vi "Response hndler.vi"(10 "Recived MSG":string, 11 "Domino LM.lvlib:Domino Laser module Class.lvclass":refnum<class "Domino Laser module Class.lvclass">) -> (1 "Command Excuted successfully?":bool, 2 "printer response":string, 3 "Domino LM.lvlib:Domino Laser module Class.lvclass 2":refnum<class "Domino Laser module Class.lvclass">)   [LabVIEW 2024, in "Domino LM.lvlib" / "Domino Laser module Class.lvclass"]
uses:
  CTRLS/Domino Laser module Class.lvclass
  <vilib>/Utility/error.llb/Trim Whitespace One-Sided.vi
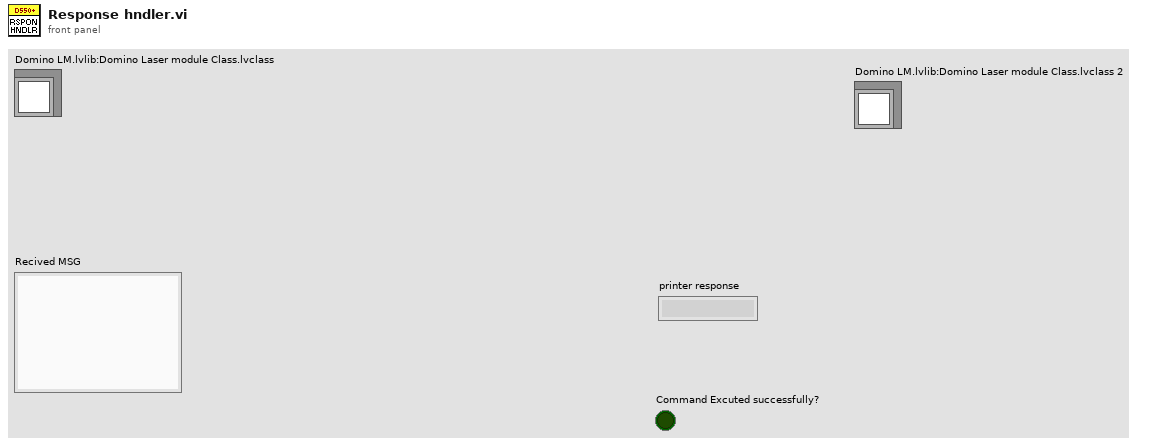
[diagram p1: front panel]
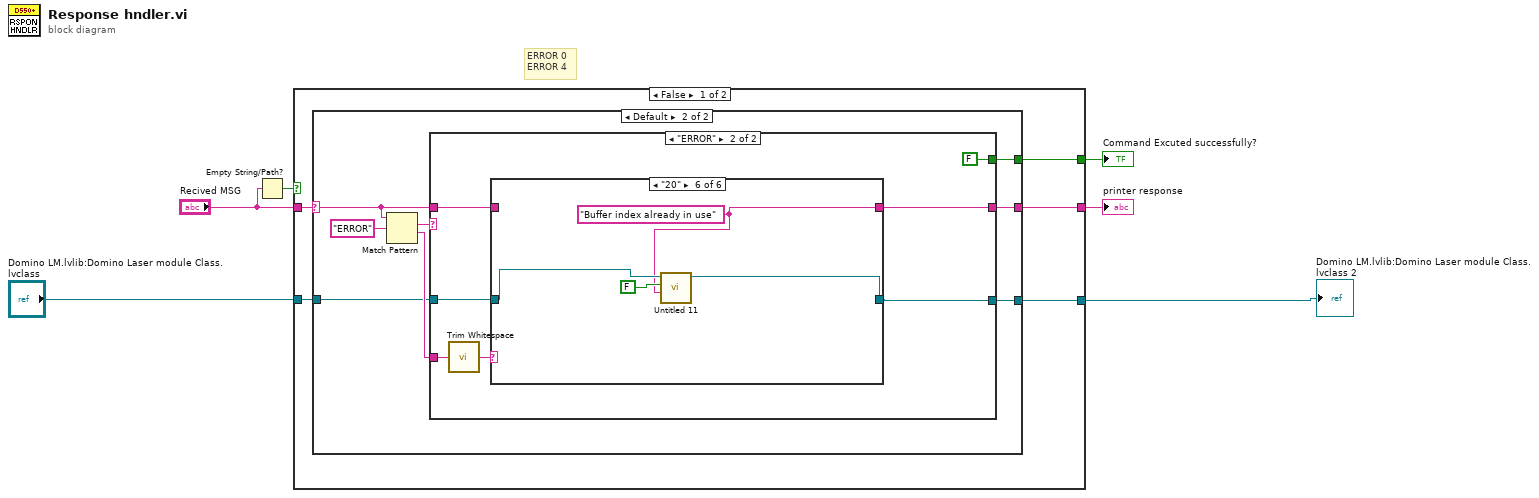
[diagram p0: block diagram]
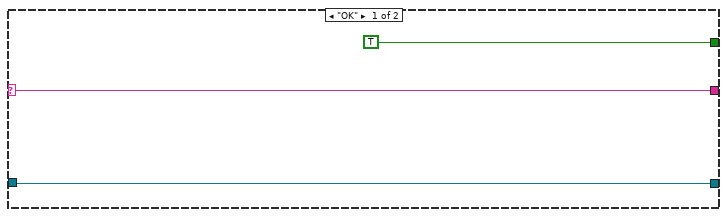
[diagram p2: hidden frame]
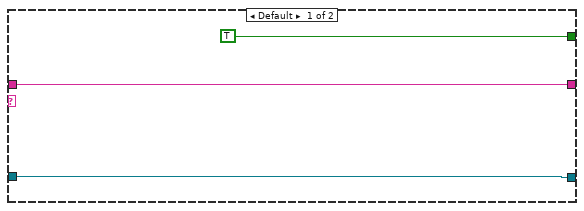
[diagram p3: hidden frame]
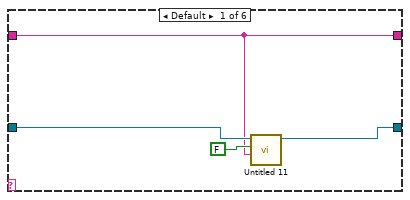
[diagram p4: hidden frame]
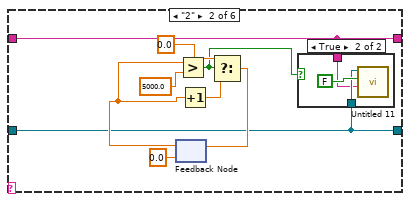
[diagram p5: hidden frame]
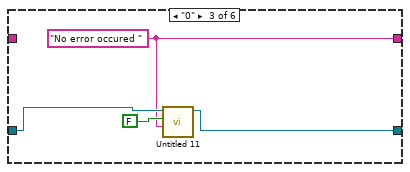
[diagram p7: hidden frame]
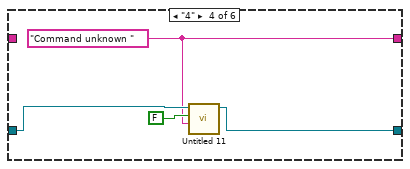
[diagram p8: hidden frame]
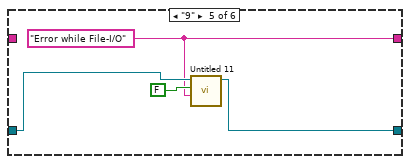
[diagram p9: hidden frame]
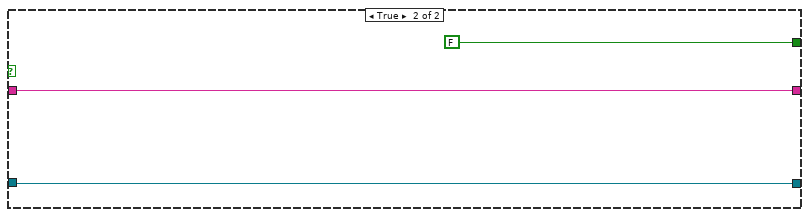
[diagram p10: hidden frame]
diagram:
  # "ERROR 0\nERROR 4"
  n1 = Empty String/Path?(string/path="Recived MSG") -> (empty?=w3:bool)
  n2 = case shown="False" w3 {
    tunnel: "Recived MSG" -> [w11 w66]
    tunnel: [w10 FALSE] -> w6
    tunnel: [w9 w66] -> w5
    tunnel: "Domino LM.lvlib:Domino Laser module Class.lvclass" -> [w8 w65]
    tunnel: [w7 w65] -> w1
    frame False {
      n3 = case shown="Default" w11 {
        selector: w11 -> [w13 w20]
        tunnel: [TRUE w17] -> w10
        tunnel: [w13 w21] -> w9
        tunnel: w8 -> [w12 w16]
        tunnel: [w12 w15] -> w7
        frame "OK" {
        }
        frame Default {
          n4 = Match Pattern(string=w20, regular expression="ERROR") -> (match substring=w18:string, after substring=w19:string)  [unwired: 1 in, 2 out]
          n5 = case shown="\"ERROR\"" w18 {
            tunnel: [w24 w27] -> w21
            tunnel: w20 -> [w24 w32]
            tunnel: w19 -> [_ w31]
            tunnel: [TRUE FALSE] -> w17
            tunnel: w16 -> [w23 w28]
            tunnel: [w23 w26] -> w15
            frame Default {
            }
            frame "ERROR" {
              n6 = call <vilib>:"Trim Whitespace.vi"("string"=w31) -> ("trimmed string"=w30:string)  [unwired: 1 in]
              n7 = case shown="\"20\"" w30 {
                tunnel: [w33 w37 w49 w53 w57 w61] -> w27
                tunnel: w32 -> [w33 w37 _ _ _ _]
                tunnel: w28 -> [w35 w38 w51 w55 w59 w63]
                tunnel: [w34 w38 w50 w54 w58 w62] -> w26
                frame Default {
                  n8 = call "Untitled 11.vi"("MSG"=w33, "MSG Status"=FALSE, "Domino Laser module Class in"=w35) -> ("Domino Laser module Class out"=w34:refnum<class "Domino Laser module Class.lvclass">)  [unwired: 7 in, 1 out]
                }
                frame "2" {
                  n9 = feedback #1(0.0 ("t")) -> (w40:dbl)
                  n10 = Greater?(x=w40, y=5000.0) -> (0:w39:bool)
                  n11 = Increment(x=w40) -> (x+1=w43:dbl)
                  n12 = Select(t=0.0, s=w39, f=w43) -> (s? t:f=w42:dbl)
                  n13 = feedback-in #1(w42) -> ()
                  n14 = case shown="True" w39 {
                    tunnel: w38 -> [_ w47]
                    tunnel: w37 -> [_ w46]
                    frame False {
                    }
                    frame True {
                      n15 = call "Untitled 11.vi"("MSG"=w46, "MSG Status"=FALSE, "Domino Laser module Class in"=w47) -> ()  [unwired: 7 in, 2 out]
                    }
                  }
                }
                frame "0" {
                  w49 = "No error occured "
                  n16 = call "Untitled 11.vi"("MSG"=w49, "MSG Status"=FALSE, "Domino Laser module Class in"=w51) -> ("Domino Laser module Class out"=w50:refnum<class "Domino Laser module Class.lvclass">)  [unwired: 7 in, 1 out]
                }
                frame "4" {
                  w53 = "Command unknown "
                  n17 = call "Untitled 11.vi"("MSG"=w53, "MSG Status"=FALSE, "Domino Laser module Class in"=w55) -> ("Domino Laser module Class out"=w54:refnum<class "Domino Laser module Class.lvclass">)  [unwired: 7 in, 1 out]
                }
                frame "9" {
                  w57 = "Error while File-I/O"
                  n18 = call "Untitled 11.vi"("MSG"=w57, "MSG Status"=FALSE, "Domino Laser module Class in"=w59) -> ("Domino Laser module Class out"=w58:refnum<class "Domino Laser module Class.lvclass">)  [unwired: 7 in, 1 out]
                }
                frame "20" {
                  w61 = "Buffer index already in use"
                  n19 = call "Untitled 11.vi"("MSG"=w61, "MSG Status"=FALSE, "Domino Laser module Class in"=w63) -> ("Domino Laser module Class out"=w62:refnum<class "Domino Laser module Class.lvclass">)  [unwired: 7 in, 1 out]
                }
              }
            }
          }
        }
      }
    }
    frame True {
    }
  }
  "Command Excuted successfully?" <- w6
  "printer response" <- w5
  "Domino LM.lvlib:Domino Laser module Class.lvclass 2" <- w1
